vi "global.vi"() -> ()   [LabVIEW 2018]
panel:
  in  "Format":cluster{"Rate":i32, "Bits":i32, "Channels":u32}={"Rate"=44100, "Bits"=32, "Channels"=2}
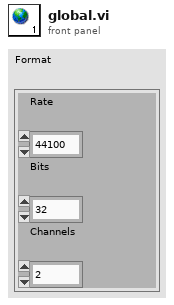
[diagram p1: front panel]
diagram:
